vi "2100_Test_Rfree_Per_Throw.vi"(0 "Semiconductor Module Context":T7, 1 "USID":T4, 2 "current range":dbl=1e-05 format="%#_6p", 3 "current level":dbl=1e-05 format="%#_13p", 5 "Script_Info":T3={"Script Name"="WalkingState", "All_Scripts"=[]}, 9 "Instrument_Pins":T6={"SMU_Pins"=["RF1", "RF2", "RF3", "RF4"], "HSDIO_Pins"=["CLK", "SDA"]}, 11 "Error In":errorcluster, 12 "Master_Register_Data_Array_In":T1 {"Address" format="%.0x"}, 13 "Reg_Map_and_Bit_Name":T5={"Reg_Map_Bit_Name"="", "Reg_Map"=[["Reg Addr(0x00)", "7", "6", "5", "4", "3", "2", "1", "0"], ["0", "SPARE", "RF3_SH", "RF2_SH", "RF1_SH", "SPARE", "RF3_RFC", "RF2_RFC", "RF1_RFC"], ["1", "SPARE[7:0]", "", "", "", "", "", "", ""], ["2", "VVAR_EN", "LCM_EN", "RFC_SH", "SPARE", "VARACTOR[3:0]", "", "", ""], ["3", "SW_CTRL1_VIRTUAL[7:0]", "", "", "", "", "", "", ""], ["4", "SW_CTRL1_SWAP", "SW_CTRL1_RBSHIFT[2:0]", "", "", "SW_CTRL1_VSID[3:0]", "", "", ""], ["5", "REG_00_VIRTUAL_MASK[7:0]", "", "", "", "", "", "", ""], ["6", "LOCK_STATUS[1:0]", "", "CLK_DITHER", "FUSES_BURNED", "CLK_IDAC_CAL[3:0]", "", "", ""], ["7", "SPARE[2:0]", "", "", "ODFT_TRIM[4:0]", "", "", "", ""], ["8", "SPARE[2:0]", "", "", "HV_TRIM[4:0]", "", "", "", ""], ["9", "TEST_MUX[2:0]", "", "", "SPARE[1:0]", "", "MEMS_BG_TC[1:0]", "", "MEMSCP_RCM"], ["A", "CP_BOOST_OVRD_EN", "SPARE[2:0]", "", "", "PS_OFF_TIMER[1:0]", "", "PS_ON_TIMER[1:0]", ""], ["0", "", "", "", "", "", "", "", ""], ["D", "Reserved[1:0]", "", "WD_HI_EVENT_CNT[5:0]", "", "", "", "", ""], ["E", "VERSION_ID[7:0]", "", "", "", "", "", "", ""], ["F", "Reserved", "COUNT_200_LSB[6:0]", "", "", "", "", "", ""], ["10", "CLK_DIV2_EN", "Spare", "ODFT_EN", "HV_HYST[4:0]", "", "", "", ""], ["0", "", "", "", "", "", "", "", ""], ["12", "SHORT_FUSE", "FUSE_BURN", "STROBE_EN", "VIO_OK", "RTH[1:0]", "", "FUSE_LOAD_MAN_EN", "FUSE_LOAD"], ["13", "RR_ACK_EN", "Reserved", "ACK_POSITION[1:0]", "", "SuBUS_DRIVE_STRENGTH[3:0]", "", "", ""], ["14", "TM_IO_EN", "TM_IO_SEL", "SuBUS_OVS[1:0]", "", "Reserved[3:0]", "", "", ""], ["15", "Reserved[4:0]", "", "", "", "", "SuBUS_VERSION_PRESENT", "SuBUS_VOLTAGE", "SuBUS_FLAVOR_DEF"], ["16", "PROG_STROBE1_DUR[7:0]", "", "", "", "", "", "", ""], ["17", "PROG_STROBE0_DUR[7:0]", "", "", "", "", "", "", ""], ["18", "Reserved[2:0]", "", "", "EFUSE_SINGLE_ADDR_SEL[4:0]", "", "", "", ""], ["19", "POLL_ADR[4:0]", "", "", "", "", "POLL_BC[2:0]", "", ""], ["1A", "SOFTWARE_RESET", "Reserved[6:0]", "", "", "", "", "", ""], ["1B", "Reserved[7:0]", "", "", "", "", "", "", ""], ["1C", "PWR_MODE_1", "PWR_MODE_0", "TRIGGER_MASK[2:0]", "", "", "TRIGGER[2:0]", "", ""], ["1D", "PRODUCT_ID[7:0]", "", "", "", "", "", "", ""], ["1E", "MANUFACTURER_ID_LSB[7:0]", "", "", "", "", "", "", ""], ["1F", "MANUFACTURER_ID_MSB[3:0]", "", "", "", "USID[3:0]", "", "", ""]]}) -> (6 "Master_Register_Data_Array_Out":T1 {"Address" format="%.0x"}, 15 "Error Out":errorcluster)   [LabVIEW 2013]
uses:
  Controls/USID.ctl
  <vilib>/NI_TestStand_SemiconductorModule/NI_TestStand_Semiconductor_Module.lvlibp/PinMap/General/SemiconductorModuleContext.ctl
  Controls/Master_Reg_Data_Array.ctl
  Controls/Reg_Address_Data.ctl
  <vilib>/NI_TestStand_SemiconductorModule/NI_TestStand_Semiconductor_Module.lvlibp/PinMap/General/Publish/PublishDataDoubleFunctionalTest.vi
  <vilib>/NI_TestStand_SemiconductorModule/NI_TestStand_Semiconductor_Module.lvlibp
panel:
  out "Data_Names":string[](array[string])
  out "Data_to_Log":dbl[](array[numeric])
  out "R_Measurements":dbl[][](array[numeric]) format="%#_6p"
  in  "Tab Control":enum32{"Test Info", "Instrument Settings"}(tab)
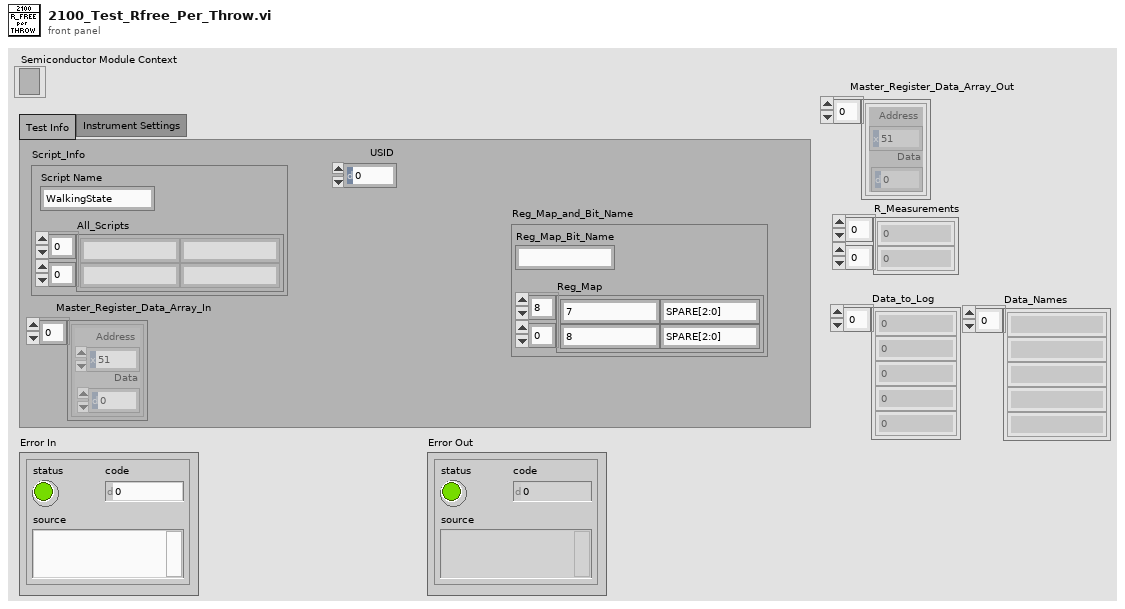
[diagram p1: front panel]
types:
  T1 = typedef "Master_Reg_Data_Array.ctl" = T2[]
  T2 = typedef "Reg_Address_Data.ctl" = cluster{"Address":u8, "Data":u8}
  T3 = cluster{"Script Name":string, "All_Scripts":string[][]}
  T4 = typedef "USID.ctl" = u8
  T5 = cluster{"Reg_Map_Bit_Name":string, "Reg_Map":string[][]}
  T6 = cluster{"SMU_Pins":string[], "HSDIO_Pins":string[]}
  T7 = typedef "NI_TestStand_Semiconductor_Module.lvlibp/SemiconductorModuleContext.ctl" = refnum<k7>
  T8 = typedef "Script Functions_Array.ctl" = enum16{"Reg_Write", "Bit_Write", "Delay", "Read", "Measure"}[]
  T9 = enum16{"Reg_Write", "Bit_Write", "Delay", "Read", "Measure"}
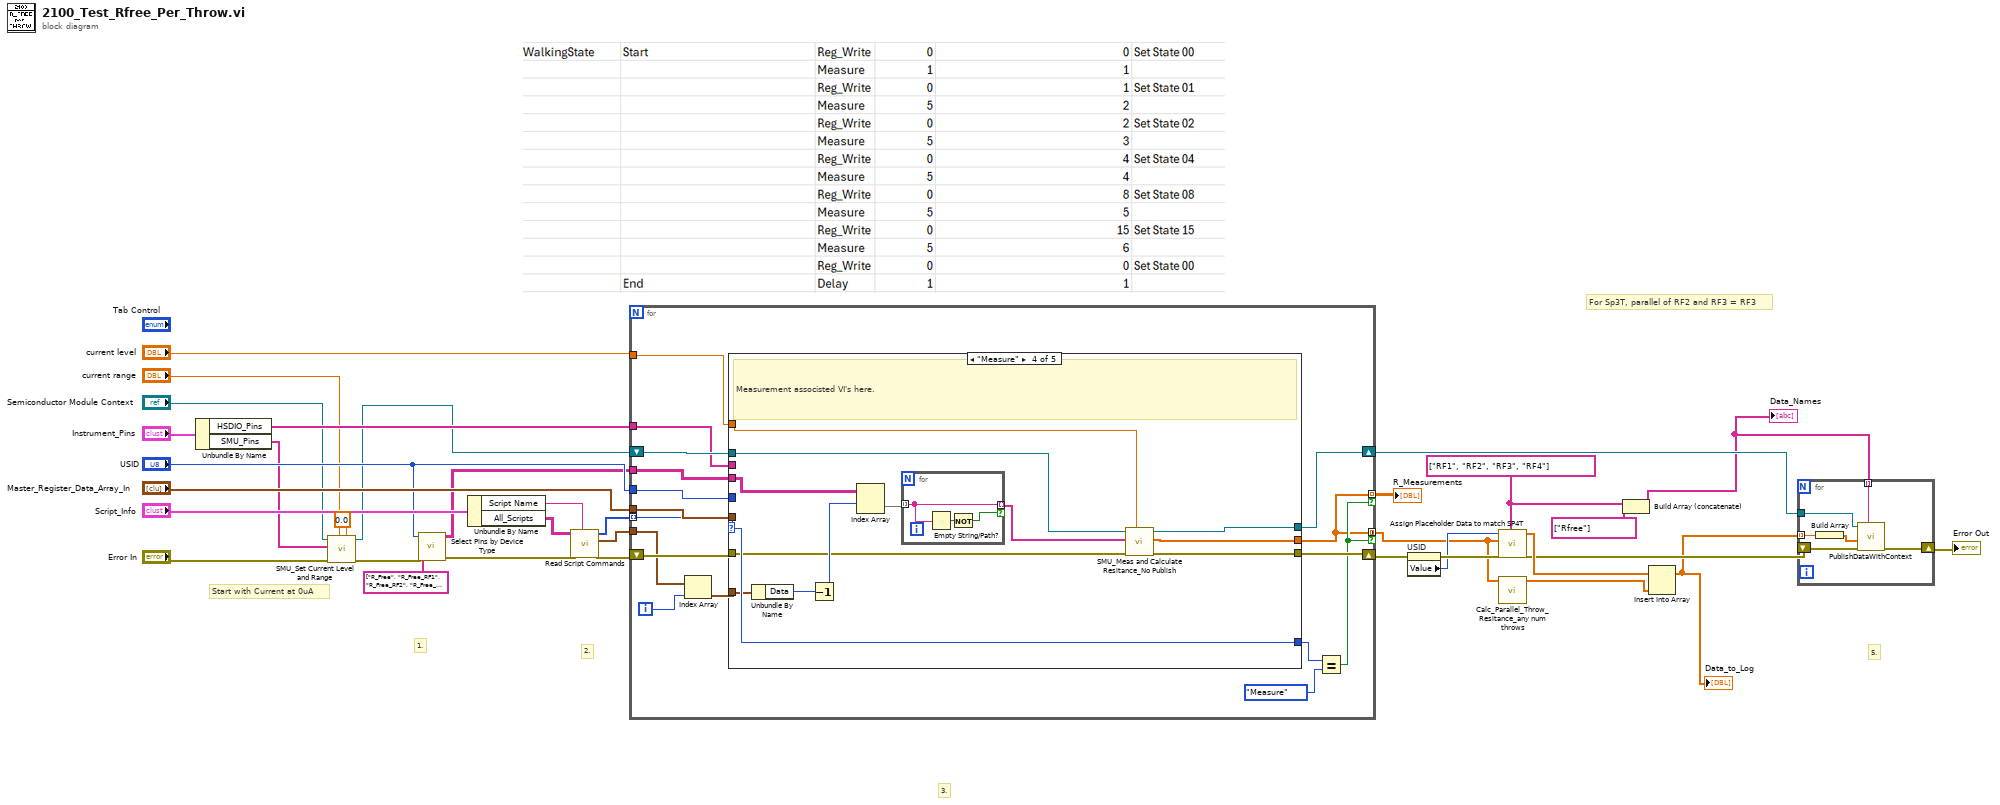
[diagram p0: block diagram]
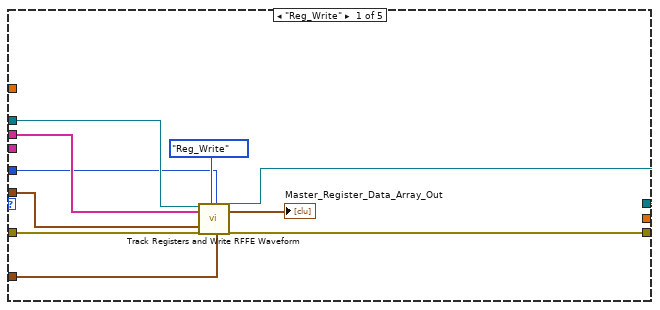
[diagram p2: hidden frame]
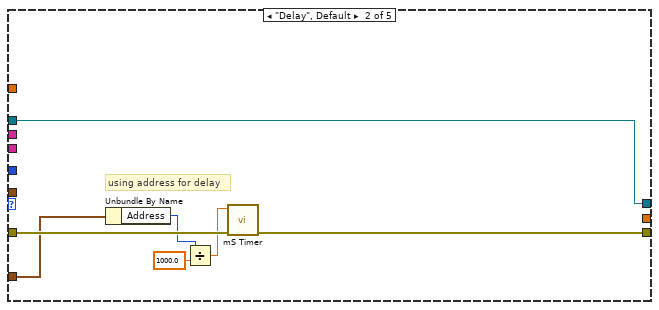
[diagram p3: hidden frame]
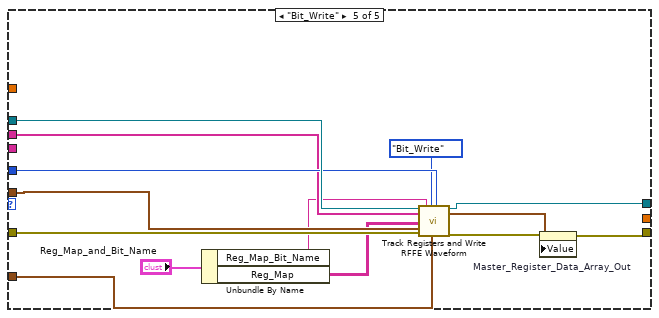
[diagram p5: hidden frame]
diagram:
  w19 = string[] ["RF1", "RF2", "RF3", "RF4"] ("SP4T_Pins")
  # "Start with Current at 0uA"
  # "For Sp3T, parallel of RF2 and RF3 = RF3"
  # "5."
  # "3."
  # "2."
  # "1."
  n1 = Unbundle By Name("Instrument_Pins") -> ("HSDIO_Pins"=w30:string[], "SMU_Pins"=w3:string[])
  n2 = call "SMU_Set Current Level and Range.vi"("current level"=0.0, "current range"="current range", "error in (no error)"="Error In", "Pins"=w3, "Semiconductor Module Context"="Semiconductor Module Context") -> ("error out"=w8:errorcluster, "Semiconductor Module Context Out"=w5:T7)  [unwired: 5 in]
  n3 = call "Select Pins by Device Type.vi"("error in (no error)"=w8, "Publishable IDs"=string[] ["R_Free", "R_Free_RF1", "R_Free_RF2", "R_Free_RF3", "R_Free_RF4"], "USID"="USID") -> ("error out"=w23:errorcluster, "Pins to Test"=w20:string[][])  [unwired: 7 in]
  n4 = Unbundle By Name("Script_Info") -> ("Script Name"=w27:string, "All_Scripts"=w28:string[][])
  n5 = call "Read Script Commands.vi"("Test Name"=w27, "Error In"=w23, "All_Scripts"=w28) -> ("Error Out"=w33:errorcluster, "Script_Data"=w34:T2[], "Script_Functions"=w35:T8)  [unwired: 5 in, 1 out]
  n6 = for {
    tunnel: "USID" -> [w46]
    tunnel: w35 -> [w45] mode=indexing
    tunnel: w34 -> [w49]
    tunnel: w30 -> [w50]
    shift-right: [w43] -> w24
    shift-left: w33 -> [w52]
    tunnel: "Master_Register_Data_Array_In" -> [w47]
    tunnel: [w37] -> w15 mode=indexing if=w38
    shift-right: [w42] -> w25
    shift-left: w5 -> [w51]
    tunnel: w20 -> [w39]
    tunnel: [w37] -> w13 mode=concatenating if=w38
    tunnel: "current level" -> [w36]
    i -> [w44]
    n7 = Index Array(array=w49, index=w44) -> (element=w48:T2)
    n8 = case shown="\"Measure\"" w45 {
      selector: w45 -> [_ _ _ w84 _]
      tunnel: w48 -> [w58 w68 _ w81 w88]
      tunnel: w52 -> [w62 w69 w71 w78 w101]
      tunnel: w46 -> [w55 _ _ _ w95]
      tunnel: w51 -> [w61 w63 w70 w76 w96]
      tunnel: w50 -> [w60 _ _ _ w93]
      tunnel: [w53 w67 w71 w75 w99] -> w43
      tunnel: w47 -> [w57 _ _ _ w92]
      tunnel: [w54 w63 w70 w74 w97] -> w42
      tunnel: [_ _ _ w84 _] -> w40
      tunnel: w39 -> [_ _ _ w79 _]
      tunnel: [_ _ _ w73 _] -> w37
      tunnel: w36 -> [_ _ _ w72 _]
      frame "Reg_Write" {
        n9 = call "Track Registers and Write RFFE Waveform.vi"("Semiconductor Module Context"=w61, "Pins"=w60, "Master_Register_Data_Array_In"=w57, "Error In"=w62, "Script_Functions"=enum16{"Reg_Write", "Bit_Write"}."Reg_Write", "USID"=w55, "Reg_Address_Data"=w58) -> ("Semiconductor Module Context Out"=w54:T7, "Master_Register_Data_Array_Out"=→"Master_Register_Data_Array_Out":T1, "Error Out"=w53:errorcluster)  [unwired: 10 in]
      }
      frame "Delay", Default {
        # "using address for delay"
        n10 = Unbundle By Name(w68) -> ("Address"=w65:u8)
        n11 = Divide(x=w65, y=1000.0) -> (x/y=w64:dbl)
        n12 = call "mS Timer.vi"("Error In"=w69, "Delay(S)"=w64) -> ("Error Out"=w67:errorcluster)  [unwired: 9 in]
      }
      frame "Read" {
        # "Future Dev Code"
      }
      frame "Measure" {
        # "Measurement associsted VI's here."
        n13 = Unbundle By Name(w81) -> ("Data"=w82:u8)
        n14 = Decrement(x=w82) -> (x-1=w80:u8)
        n15 = Index Array(array=w79, index (row)=w80) -> (element=w83:string[])  [unwired: 1 in]
        n16 = for {
          tunnel: w83 -> [w87] mode=indexing
          tunnel: [w87] -> w77 mode=indexing if=w85
          n17 = Empty String/Path?(string/path=w87) -> (empty?=w86:bool)
          n18 = Not(x=w86) -> (.not. x?=w85:bool)
        }
        n19 = call "SMU_Meas and Calculate Resitance_No Publish.vi"("Current  Level"=w72, "error in (no error)"=w78, "Pins"=w77, "Semiconductor Module Context"=w76) -> ("error Out"=w75:errorcluster, "R Array"=w73:dbl[], "Semiconductor Module Context Out"=w74:T7)  [unwired: 4 in, 1 out]
      }
      frame "Bit_Write" {
        n20 = Unbundle By Name("Reg_Map_and_Bit_Name") -> ("Reg_Map_Bit_Name"=w90:string, "Reg_Map"=w89:string[][])
        n21 = call "Track Registers and Write RFFE Waveform.vi"("Semiconductor Module Context"=w96, "Pins"=w93, "Reg_Map"=w89, "Master_Register_Data_Array_In"=w92, "Error In"=w101, "Reg_Map_Bit_Name"=w90, "Script_Functions"=enum16{"Reg_Write", "Bit_Write"}."Bit_Write", "USID"=w95, "Reg_Address_Data"=w88) -> ("Semiconductor Module Context Out"=w97:T7, "Master_Register_Data_Array_Out"=w98:T1, "Error Out"=w100:errorcluster)  [unwired: 8 in]
        n22 = property on="Master_Register_Data_Array_Out" class="Arr (strict)"(error in=w100, "Value"=w98) -> (error out=w99:errorcluster)  [unwired: 1 in, 1 out]
      }
    }
    n23 = Equal?(x=w40, y=T9."Measure" ("Enum")) -> (x = y?=w38:bool)
  }
  "R_Measurements" <- w15
  n24 = property on="USID" class="DigNum (strict)"(error in=w24) -> (error out=w17:errorcluster, "Value"=w16:T4)  [unwired: 1 in, 1 out]
  n25 = call "Assign Placeholder Data to match SP4T.vi"("SP4T_Pins"=w19, "error in (no error)"=w17, "Individual_R_Meas"=w13, "USID"=w16) -> ("error out"=w11:errorcluster, "Placeholder_w_Data"=w14:dbl[])  [unwired: 6 in]
  n26 = call "Calc_Parallel_Throw_Resitance_any num throws.vi"("Resitance_Per Site"=w13) -> ("Parallel_Resitance"=w12:dbl[])  [unwired: 10 in]
  n27 = Build Array (concatenate)(w19, string[] ["Rfree"] ("element")) -> (w9:string[])
  "Data_Names" <- w9
  n28 = Insert Into Array(array=w14, new element=w12) -> (w10:dbl[])  [unwired: 1 in]
  "Data_to_Log" <- w10
  n29 = for {
    shift-right: [w107] -> w26
    shift-left: w11 -> [w106]
    tunnel: w25 -> [w105]
    tunnel: w10 -> [w104] mode=indexing
    tunnel: w9 -> [w102] mode=indexing
    n30 = Build Array(w104) -> (w103:dbl[])
    n31 = call-poly <vilib>:"PublishDataWithContext.vi"("Published Data Id"=w102, "error in (no error)"=w106, "Data In"=w103, "Semiconductor Module Context"=w105) -> ("error out"=w107:errorcluster)  [unwired: 6 in, 1 out]
  }
  "Error Out" <- w26
